vi "Get_Parent_Applies.vi"(8 "error in (no error)":errorcluster, 11 "AB_Source_Container in":refnum<class "AB_Source_Container.lvclass">) -> (0 "error out":errorcluster, 2 "parentApplies":T1, 3 "AB_Source_Container out":refnum<class "AB_Source_Container.lvclass">)   [LabVIEW 2020, in "AB_Source_Container.lvclass"]
uses:
  <vilib>/AppBuilder/AB_Classes/Source/Container/AB_Source_Container.lvclass
  <vilib>/AppBuilder/AB_Parent_Applies.ctl
  <vilib>/AppBuilder/AB_Classes/Source/Container/AB_Source_Container.lvclass/AB_Source_Container.ctl
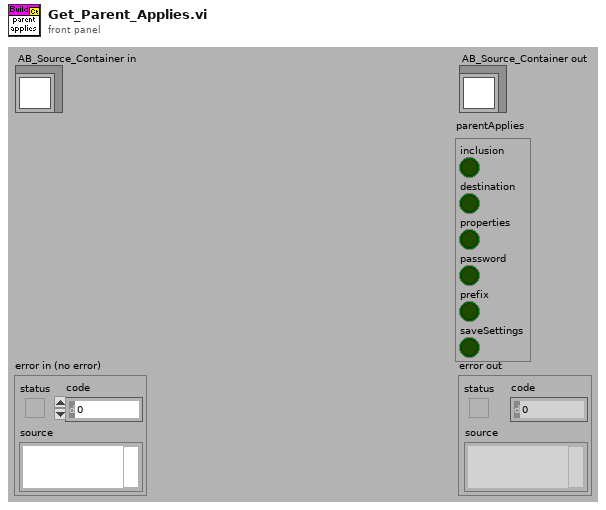
[diagram p1: front panel]
types:
  T1 = typedef "AB_Parent_Applies.ctl" = cluster{"inclusion":bool, "destination":bool, "properties":bool, "password":bool, "prefix":bool, "saveSettings":bool}
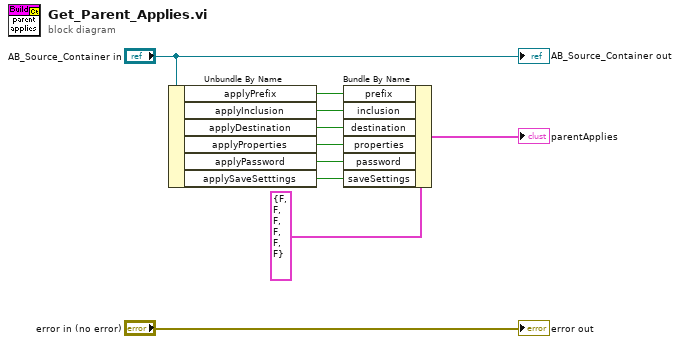
[diagram p0: block diagram]
diagram:
  n1 = Unbundle By Name("AB_Source_Container in") -> ("applyPrefix"=w2:bool, "applyInclusion"=w7:bool, "applyDestination"=w6:bool, "applyProperties"=w5:bool, "applyPassword"=w4:bool, "applySaveSetttings"=w3:bool)
  n2 = Bundle By Name(cluster=T1 {"inclusion"=FALSE, "destination"=FALSE, "properties"=FALSE, "password"=FALSE, "prefix"=FALSE, "saveSettings"=FALSE} ("parentApplies"), "prefix"=w2, "inclusion"=w7, "destination"=w6, "properties"=w5, "password"=w4, "saveSettings"=w3) -> (→"parentApplies":T1)
  "error out" <- "error in (no error)"
  "AB_Source_Container out" <- "AB_Source_Container in"
